vi "populate sonde row cluster.vi"(7 "Initialize Initial Value Cluster":bool, 8 "error in (no error)":errorcluster, 9 "Sonde Parameters \nInitial Values":T1 {"Salinity Initial" format="%_2f"; "Temp Initial" format="%_2f"; "ORP  Initial" format="%_2f"; "pH Initial" format="%_2f"; "DO Initial" format="%_2f"; "SC Initial" format="%_2f"}, 10 "Array In":string[](array[string]), 11 "Sonde Parameters \nTolerance Limits":T4 {"Salinity %" format="%_2f%%"; "Temp %" format="%_2f%%"; "ORP %" format="%_2f%%"; "pH %" format="%_2f%%"; "DO %" format="%_2f%%"; "SC %" format="%_2f%%"}) -> (0 "error out":errorcluster, 1 "Cluster":T2 {"Salinity"."%" format="%_2f%%"; "Salinity"."Value" format="%_4g"; "Temperature"."%" format="%_2f%%"; "Temperature"."Value" format="%_4g"; "ORP"."%" format="%_2f%%"; "ORP"."Value" format="%_4g"; "pH"."%" format="%_2f%%"; "pH"."Value" format="%_4g"; "Dissolved Oxygen"."%" format="%_2f%%"; "Dissolved Oxygen"."Value" format="%_4g"; "Sp. Conductance"."%" format="%_2f%%"; "Sp. Conductance"."Value" format="%_4g"; "Cumulative\nVolume" format="%#_4g"}, 2 "Time Value":dbl, 3 "Array out":string[](array[string]), 6 "Sonde Parameters \nInitial Values Out":T1 {"Salinity Initial" format="%_2f"; "Temp Initial" format="%_2f"; "ORP  Initial" format="%_2f"; "pH Initial" format="%_2f"; "DO Initial" format="%_2f"; "SC Initial" format="%_2f"})   [LabVIEW 2016]
uses:
  activeXtest/activeXtest 2015 Folder/sonde cluster from excel.ctl
  Sonde Value Percent Tol.ctl
panel:
  in  "Input Cluster for % calculation":T2 caption="Cluster" {"Salinity"."%" format="%_2f%%"; "Salinity"."Value" format="%_4g"; "Temperature"."%" format="%_2f%%"; "Temperature"."Value" format="%_4g"; "ORP"."%" format="%_2f%%"; "ORP"."Value" format="%_4g"; "pH"."%" format="%_2f%%"; "pH"."Value" format="%_4g"; "Dissolved Oxygen"."%" format="%_2f%%"; "Dissolved Oxygen"."Value" format="%_4g"; "Sp. Conductance"."%" format="%_2f%%"; "Sp. Conductance"."Value" format="%_4g"; "Cumulative\nVolume" format="%#_4g"}
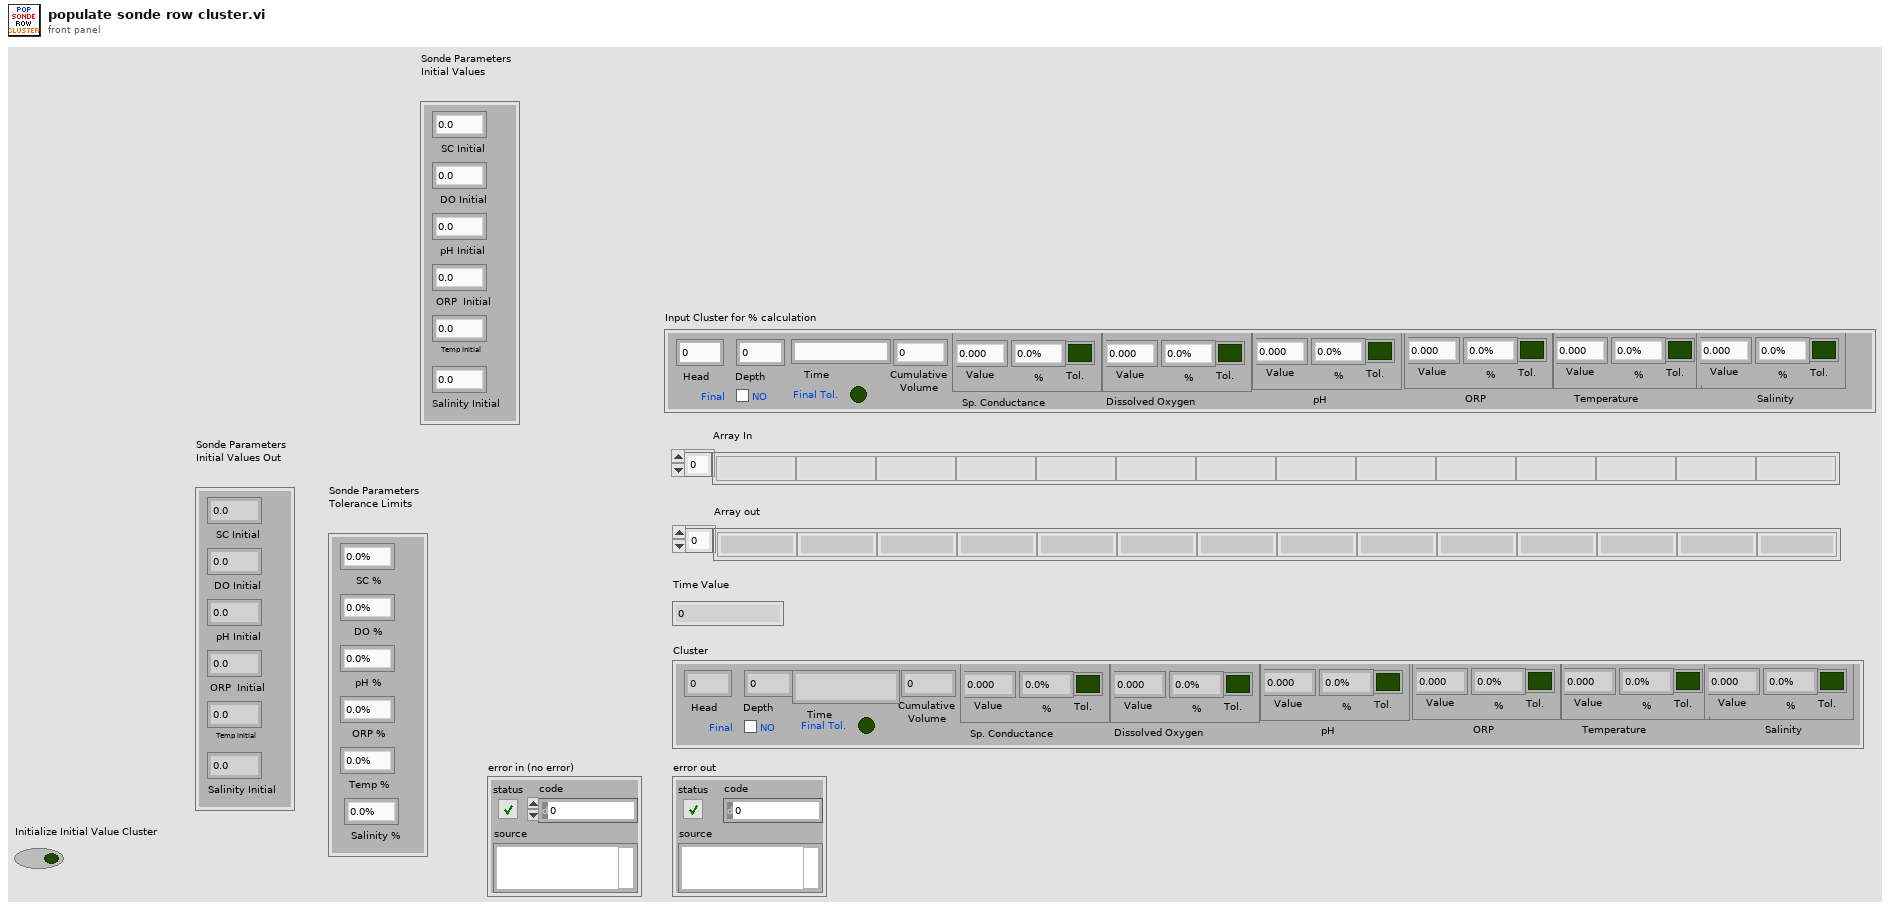
[diagram p1: front panel]
types:
  T1 = cluster{"SC Initial ":dbl, "DO Initial ":dbl, "pH Initial  ":dbl, "ORP  Initial":dbl, "Temp Initial":dbl, "Salinity Initial ":dbl}
  T2 = typedef "sonde cluster from excel.ctl" = cluster{"Head":dbl, "Depth":dbl, "Time":string, "Cumulative\nVolume":dbl, "Sp. Conductance":T3, "Dissolved Oxygen":T3, "pH":T3, "ORP":T3, "Temperature":T3, "Salinity":T3, "Final Tol.":bool, "Final":bool}
  T3 = typedef "Sonde Value Percent Tol.ctl" = cluster{"Value":dbl, "%":dbl, "Tol.":bool}
  T4 = cluster{"SC %":dbl, "DO %":dbl, "pH % ":dbl, "ORP % ":dbl, "Temp % ":dbl, "Salinity %":dbl}
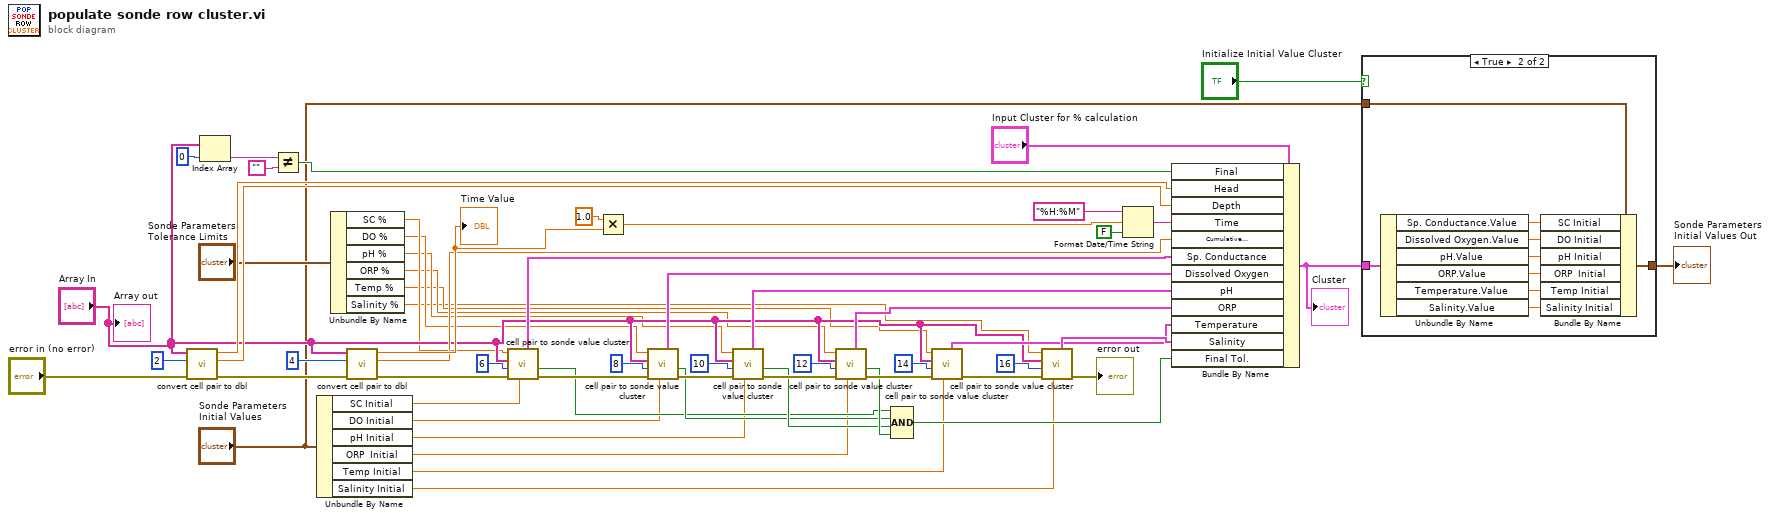
[diagram p0: block diagram]
diagram:
  n1 = call "convert cell pair to dbl.vi"("error in"="error in (no error)", "start index"=2 ("index"), "Array"="Array In") -> ("error out"=w56:errorcluster, "Numeric of start index +1"=w29:dbl, "Numeric of start index"=w28:dbl)  [unwired: 6 in]
  n2 = Index Array(array="Array In", index=0) -> (element=w59:string)
  n3 = Not Equal?(x=w59, y="") -> (x != y?=w22:bool)
  n4 = Unbundle By Name("Sonde Parameters \nInitial Values") -> ("SC Initial"=w9:dbl, "DO Initial"=w8:dbl, "pH Initial"=w7:dbl, "ORP  Initial"=w6:dbl, "Temp Initial"=w5:dbl, "Salinity Initial"=w4:dbl)
  n5 = Unbundle By Name("Sonde Parameters \nTolerance Limits") -> ("SC %"=w19:dbl, "DO %"=w18:dbl, "pH %"=w17:dbl, "ORP %"=w16:dbl, "Temp %"=w15:dbl, "Salinity %"=w14:dbl)
  n6 = call "convert cell pair to dbl.vi"("error in"=w56, "start index"=4, "Array"="Array In") -> ("error out"=w55:errorcluster, "Numeric of start index +1"=w31:dbl, "Numeric of start index"=w58:dbl)  [unwired: 6 in]
  "Time Value" <- w58
  n7 = call "cell pair to sonde value cluster.vi"("Initial Value"=w9, "error in"=w55, "start index"=6, "Array"="Array In", "tolerance limit"=w19) -> ("error out"=w54:errorcluster, "Tolerance"=w43:bool, "Cluster Out"=w33:T3)  [unwired: 2 in, 2 out]
  n8 = Multiply(x=1.0, y=w58) -> (x*y=w13:dbl)
  n9 = call "cell pair to sonde value cluster.vi"("Initial Value"=w8, "error in"=w54, "start index"=8 ("index"), "Array"="Array In", "tolerance limit"=w18) -> ("error out"=w53:errorcluster, "Tolerance"=w44:bool, "Cluster Out"=w34:T3)  [unwired: 2 in, 2 out]
  n10 = call "cell pair to sonde value cluster.vi"("Initial Value"=w7, "error in"=w53, "start index"=10 ("index"), "Array"="Array In", "tolerance limit"=w17) -> ("error out"=w52:errorcluster, "Tolerance"=w45:bool, "Cluster Out"=w39:T3)  [unwired: 2 in, 2 out]
  n11 = call "cell pair to sonde value cluster.vi"("Initial Value"=w6, "error in"=w52, "start index"=12, "Array"="Array In", "tolerance limit"=w16) -> ("error out"=w51:errorcluster, "Tolerance"=w46:bool, "Cluster Out"=w40:T3)  [unwired: 2 in, 2 out]
  n12 = Compound Arithmetic op=AND(w43, w44, w45, w46) -> (w47:bool)
  n13 = call "cell pair to sonde value cluster.vi"("Initial Value"=w5, "error in"=w51, "start index"=14, "Array"="Array In", "tolerance limit"=w15) -> ("error out"=w50:errorcluster, "Cluster Out"=w41:T3)  [unwired: 2 in, 3 out]
  n14 = call "cell pair to sonde value cluster.vi"("Initial Value"=w4, "error in"=w50, "start index"=16, "Array"="Array In", "tolerance limit"=w14) -> ("error out"=→"error out":errorcluster, "Cluster Out"=w42:T3)  [unwired: 2 in, 3 out]
  n15 = Format Date/Time String(time format string (%c)="%H:%M", seconds (now)=w13, UTC format=FALSE) -> (date/time string=w25:string)
  n16 = Bundle By Name(cluster="Input Cluster for % calculation", "Final"=w22, "Head"=w28, "Depth"=w29, "Time"=w25, "Cumulative\nVolume"=w31, "Sp. Conductance"=w33, "Dissolved Oxygen"=w34, "pH"=w39, "ORP"=w40, "Temperature"=w41, "Salinity"=w42, "Final Tol."=w47) -> (w1:T2)
  "Cluster" <- w1
  n17 = case shown="True" "Initialize Initial Value Cluster" {
    tunnel: "Sonde Parameters \nInitial Values" -> [w61 w70]
    tunnel: [w61 w69] -> w3
    tunnel: w1 -> [_ w68]
    frame False {
    }
    frame True {
      n18 = Unbundle By Name(w68) -> ("Sp. Conductance.Value"=w67:dbl, "Dissolved Oxygen.Value"=w66:dbl, "pH.Value"=w65:dbl, "ORP.Value"=w64:dbl, "Temperature.Value"=w63:dbl, "Salinity.Value"=w62:dbl)
      n19 = Bundle By Name(cluster=w70, "SC Initial"=w67, "DO Initial"=w66, "pH Initial"=w65, "ORP  Initial"=w64, "Temp Initial"=w63, "Salinity Initial"=w62) -> (w69:T1)
    }
  }
  "Sonde Parameters \nInitial Values Out" <- w3
  "Array out" <- "Array In"
